vi "Write Fast FPGA Telem to TDMS.vi"   [LabVIEW 2014]
uses:
  FPGA Telem for Fast Logging.ctl
  Global Data.vi
types:
  T1 = enum16{"open", "open or create", "create or replace", "create", "open (read-only)"}
  T2 = cluster{"read mode":enum16{"polling", "blocking"}, "write mode":enum16{"polling", "blocking"}}
  T3 = typedef "FPGA Telem for Fast Logging.ctl" = cluster{"Throttle 1 (V)":fxp<+/-,24,5>, "Throttle 2 (V)":fxp<+/-,24,5>, "Throttle 1 (%)":fxp<+/-,27,18>, "Throttle 2 (%)":fxp<+/-,27,18>, "Front BP (psi)":fxp<+/-,27,16>, "Rear BP (psi)":fxp<+/-,27,16>, "Front BP (V)":fxp<+/-,24,5>, "Rear BP (V)":fxp<+/-,24,5>, "Time Stamp":timestamp, "Accel X":dbl, "Accel Y":dbl, "Accel Z":dbl, "Gyro X":dbl, "Gyro Y":dbl, "Gyro Z":dbl, "RL Tick Period":u32, "RR Tick Period":u32, "FR Tick Period":u32, "FL Tick Period":u32}
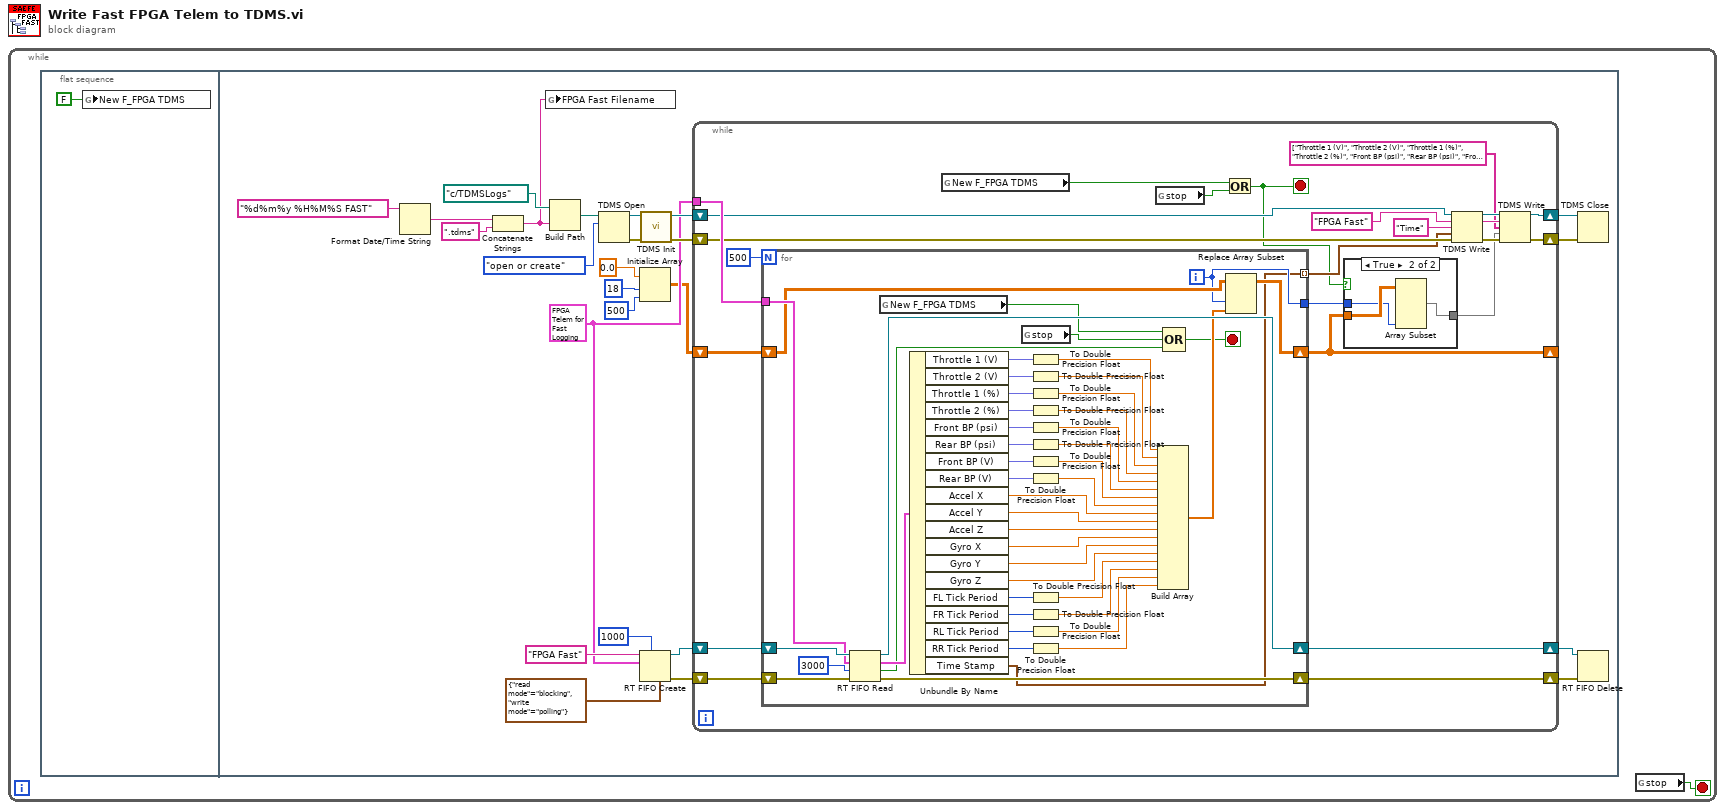
[diagram p0: block diagram]
diagram:
  n1 = while {
    stop <- w1 stop-if-true
    n2 = flat-sequence {
      frame #0 {
        n3 = global write "Global Data.vi" "New F_FPGA TDMS"(FALSE ("New F_FPGA TDMS")) -> ()
      }
      frame #1 {
        w8 = T3 {"Throttle 1 (V)"=0.4218330383300781, "Throttle 2 (V)"=0.6996517181396484, "Throttle 1 (%)"=0.0, "Throttle 2 (%)"=0.0078125, "Front BP (psi)"=186.34033203125, "Rear BP (psi)"=185.44775390625, "Front BP (V)"=0.4808177947998047, "Rear BP (V)"=0.4820976257324219, "Time Stamp"=timestamp(0 s since 1904-01-01), "Accel X"=0.0, "Accel Y"=0.0, "Accel Z"=0.0, "Gyro X"=0.0, "Gyro Y"=0.0, "Gyro Z"=0.0, "RL Tick Period"=0, "RR Tick Period"=0, "FR Tick Period"=0, "FL Tick Period"=0} ("FPGA Fast Telem")
        n4 = Format Date/Time String(time format string (%c)="%d%m%y %H%M%S FAST") -> (date/time string=w20:string)  [unwired: 2 in]
        n5 = Concatenate Strings(w20, ".tdms" ("string")) -> (w3:string)
        n6 = global write "Global Data.vi" "FPGA Fast Filename"(w3) -> ()
        n7 = Build Path(base path=path "c:/TDMSLogs", name or relative path=w3) -> (appended path=w21:path)
        n8 = TDMS Open(10:T1."open or create" ("operation (0:open)"), 11:w21) -> (0:w13:errorcluster, 3:w14:refnum<k34>)  [unwired: 5 in]
        n9 = Initialize Array(0.0 ("element"), 18 ("dimension size"), 500 ("dimension size")) -> (w4:dbl[][])
        n10 = RT FIFO Create(0:"FPGA Fast" ("name (unnamed)"), 1:w8, 4:u32 1000 ("size (10)"), 7:T2 {"read mode"=enum."blocking", "write mode"=enum."polling"} ("r/w modes (polling,polling)")) -> (8:w24:refnum<k33>, 11:w23:errorcluster)  [unwired: 4 in, 1 out]
        n11 = call "TDMS Init.vi"("error in (no error)"=w13, "tdms file"=w14) -> ("error out"=w11:errorcluster, "tdms file out"=w12:refnum<k34>)  [unwired: 8 in]
        n12 = while {
          tunnel: w8 -> [w48]
          shift-right: [w47] -> w9
          shift-left: w24 -> [w50]
          shift-right: [w46] -> w10
          shift-left: w23 -> [w49]
          shift-right: [w36] -> w16
          shift-left: w12 -> [w45]
          shift-right: [w35] -> w15
          shift-left: w11 -> [w44]
          shift-right: [w30] -> _
          shift-left: w4 -> [w34]
          stop <- w28 stop-if-true
          n13 = for {
            N: 500 -> [_]
            tunnel: w48 -> [w99]
            shift-right: [w97] -> w47
            shift-left: w50 -> [w101]
            shift-right: [w96] -> w46
            shift-left: w49 -> [w100]
            tunnel: [w64] -> w43 mode=indexing
            shift-right: [w76] -> w30
            shift-left: w34 -> [w77]
            tunnel: [w75] -> w29
            i -> [w75]
            stop <- w72 stop-if-true
            n14 = RT FIFO Read(0:w101, 1:w99, 2:3000 ("timeout in ms (0)"), 3:w100) -> (8:w97:refnum<k33>, 9:w95:T3, 10:w71:bool, 11:w96:errorcluster)  [unwired: 1 out]
            n15 = global read "Global Data.vi" "New F_FPGA TDMS"() -> (w74:bool)
            n16 = Unbundle By Name(w95) -> ("Throttle 1 (V)"=w94:fxp<+/-,24,5>, "Throttle 2 (V)"=w93:fxp<+/-,24,5>, "Throttle 1 (%)"=w92:fxp<+/-,27,18>, "Throttle 2 (%)"=w91:fxp<+/-,27,18>, "Front BP (psi)"=w90:fxp<+/-,27,16>, "Rear BP (psi)"=w89:fxp<+/-,27,16>, "Front BP (V)"=w88:fxp<+/-,24,5>, "Rear BP (V)"=w87:fxp<+/-,24,5>, "Accel X"=w70:dbl, "Accel Y"=w69:dbl, "Accel Z"=w68:dbl, "Gyro X"=w67:dbl, "Gyro Y"=w66:dbl, "Gyro Z"=w65:dbl, "FL Tick Period"=w63:u32, "FR Tick Period"=w62:u32, "RL Tick Period"=w61:u32, "RR Tick Period"=w60:u32, "Time Stamp"=w64:timestamp)
            n17 = global read "Global Data.vi" "stop"() -> (w73:bool)
            n18 = To Double Precision Float(number=w94) -> (double precision float=w86:dbl)
            n19 = To Double Precision Float(number=w93) -> (double precision float=w85:dbl)
            n20 = To Double Precision Float(number=w92) -> (double precision float=w84:dbl)
            n21 = To Double Precision Float(number=w91) -> (double precision float=w83:dbl)
            n22 = To Double Precision Float(number=w90) -> (double precision float=w82:dbl)
            n23 = To Double Precision Float(number=w89) -> (double precision float=w81:dbl)
            n24 = To Double Precision Float(number=w88) -> (double precision float=w80:dbl)
            n25 = To Double Precision Float(number=w87) -> (double precision float=w79:dbl)
            n26 = To Double Precision Float(number=w63) -> (double precision float=w59:dbl)
            n27 = To Double Precision Float(number=w62) -> (double precision float=w58:dbl)
            n28 = To Double Precision Float(number=w61) -> (double precision float=w57:dbl)
            n29 = To Double Precision Float(number=w60) -> (double precision float=w56:dbl)
            n30 = Build Array(w86, w85, w84, w83, w82, w81, w80, w79, w70, w69, w68, w67, w66, w65, w59, w58, w57, w56) -> (w78:dbl[])
            n31 = Compound Arithmetic op=OR(w74, w73, w71) -> (w72:bool)
            n32 = Replace Array Subset(array=w77, new element=w78, index (col)=w75) -> (w76:dbl[][])  [unwired: 1 in]
          }
          n33 = global read "Global Data.vi" "New F_FPGA TDMS"() -> (w32:bool)
          n34 = global read "Global Data.vi" "stop"() -> (w33:bool)
          n35 = Or(x=w32, y=w33) -> (x .or. y?=w28:bool)
          n36 = case shown="True" w28 {
            tunnel: w30 -> [w52 w55]
            tunnel: [w52 w53] -> w31
            tunnel: w29 -> [_ w54]
            frame False {
            }
            frame True {
              n37 = Array Subset(array=w55, length (col)=w54) -> (w53:dbl[][])  [unwired: 3 in]
            }
          }
          n38 = TDMS Write(0:w45, 5:"FPGA Fast" ("group name in (Untitled)"), 7:"Time", 9:w43, 11:w44) -> (4:w40:refnum<k34>, 6:w38:string, 15:w39:errorcluster)  [unwired: 1 in, 1 out]
          n39 = TDMS Write(0:w40, 5:w38, 7:string[] ["Throttle 1 (V)", "Throttle 2 (V)", "Throttle 1 (%)", "Throttle 2 (%)", "Front BP (psi)", "Rear BP (psi)", "Front BP (V)", "Rear BP (V)", "Accel X", "Accel Y", "Accel Z", "Gyro X", "Gyro Y", "Gyro Z", "FL Tick Period", "FR Tick Period", "RL Tick Period", "RR Tick Period"] ("channel name(s) in (Untitled)"), 9:w31, 11:w39) -> (4:w36:refnum<k34>, 15:w35:errorcluster)  [unwired: 1 in, 2 out]
        }
        n40 = TDMS Close(8:w15, 11:w16) -> ()  [unwired: 2 out]
        n41 = RT FIFO Delete(0:w9, 3:w10) -> ()  [unwired: 1 in, 1 out]
      }
    }
    n42 = global read "Global Data.vi" "stop"() -> (w1:bool)
  }
